vi "getBoundsRect.vi"(6 "useControlBodyOnly":bool, 8 "error in (no error)":errorcluster, 11 "ref":refnum<vi>) -> (0 "error out":errorcluster, 2 "rect":T1, 3 "ref(dup)":refnum<vi>)   [LabVIEW 2023]
doc: "Returns the bounding rectangle (Top, Left, Bottom, Right) of the input control.\nCaptions and labels are included or excluded according to the 'useControlBodyOnly' setting."
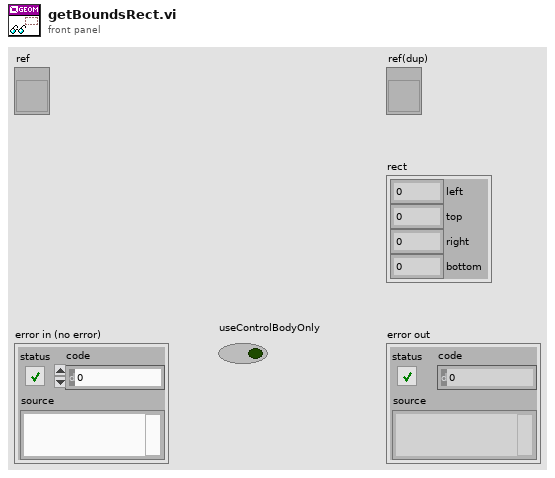
[diagram p1: front panel]
types:
  T1 = cluster{"left":i32, "top":i32, "right":i32, "bottom":i32}
  T2 = typedef "LVPositionTypeDef.ctl" = cluster{"Left":i32, "Top":i32}
  T3 = typedef "LVBoundsTypeDef.ctl" = cluster{"Width":u32, "Height":u32}
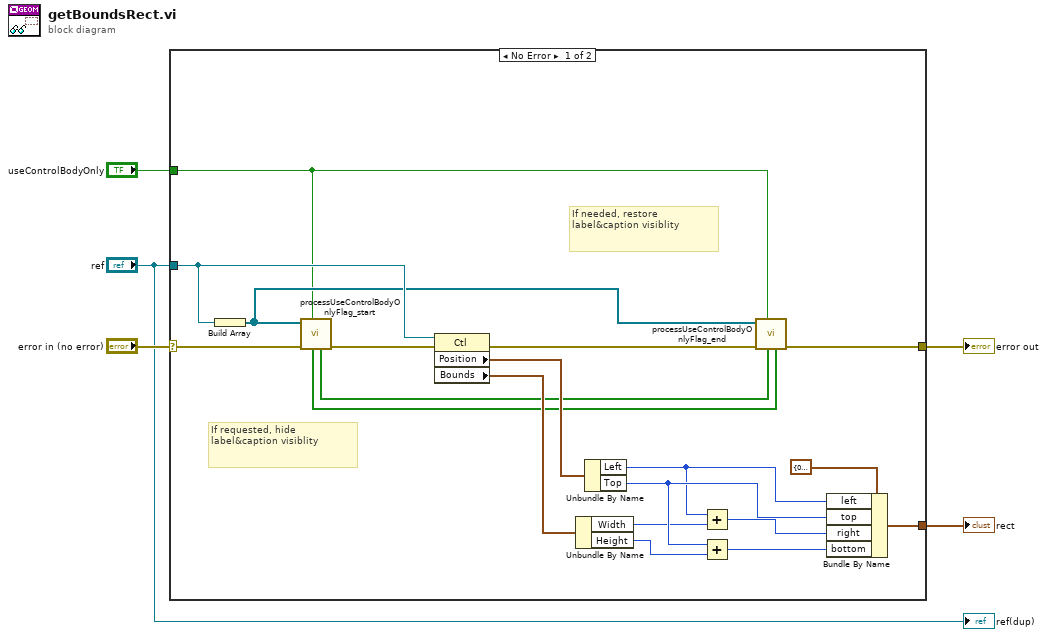
[diagram p0: block diagram]
diagram:
  n1 = case shown="No Error" "error in (no error)" {
    selector: "error in (no error)" -> [w14 w25]
    tunnel: [w24 _] -> w5
    tunnel: [w10 w25] -> w4
    tunnel: "ref" -> [w12 _]
    tunnel: "useControlBodyOnly" -> [w8 _]
    frame No Error {
      # "If needed, restore label&caption visiblity"
      # "If requested, hide label&caption visiblity"
      n2 = Build Array(w12) -> (w9:refnum<vi>[])
      n3 = call "processUseControlBodyOnlyFlag_start.vi"("useControlBodyOnly"=w8, "error in (no error)"=w14, "refList"=w9) -> ("error out"=w13:errorcluster, "LabelVisibilityList"=w7:bool[], "captionVisibilityList"=w6:bool[])  [unwired: 5 in, 1 out]
      n4 = property class="Ctl"(reference=w12, error in=w13) -> (error out=w11:errorcluster, "Position"=w16:T2, "Bounds"=w17:T3)  [unwired: 1 out]
      n5 = Unbundle By Name(w17) -> ("Width"=w19:u32, "Height"=w22:u32)
      n6 = Unbundle By Name(w16) -> ("Left"=w18:i32, "Top"=w21:i32)
      n7 = Add(x=w18, y=w19) -> (x+y=w20:u32)
      n8 = Add(x=w21, y=w22) -> (x+y=w23:u32)
      n9 = call "processUseControlBodyOnlyFlag_end.vi"("captionVisibilityList"=w6, "LabelVisibilityList"=w7, "useControlBodyOnly"=w8, "error in (no error)"=w11, "refList"=w9) -> ("error out"=w10:errorcluster)  [unwired: 5 in, 1 out]
      n10 = Bundle By Name(cluster=T1 {"left"=0, "top"=0, "right"=0, "bottom"=0} ("rect"), "left"=w18, "top"=w21, "right"=w20, "bottom"=w23) -> (w24:T1)
    }
    frame Error {
    }
  }
  "rect" <- w5
  "error out" <- w4
  "ref(dup)" <- "ref"
